vi "Puncta_fit.vi"() -> ()   [LabVIEW 2012]
uses:
  <vilib>/Utility/file.llb/Write To Spreadsheet File (DBL).vi
panel:
  in  "Batch Fit - Interate":i32=2
  in  "Reverse Order?":bool=TRUE
  in  "Single Fit":bool
  in  "Transfer to Save Buffer":bool
  out "Save Buffer":dbl[][](array[numeric])
  in  "Inverse Image?":bool=TRUE
  in  "initial parameters":dbl[](array[numeric])=[200.0, 100.0, 10.0, 10.0, 5.0, 5.0, 0.0]
  in  "Flip Width/Length?":bool=TRUE
  out "XY Fits":dbl[][](array[numeric])
  out "range fit":dbl[][](array[numeric])
  in  "Slide":cluster{i16, i16, i16}(slide)={24, 31, 24} scale=0.0..173.0
  out "Array 3":u16[][][](array[numeric])
  in  "File Path":path
  in  "Data in IFD\n(small files)":bool=TRUE
  in  "last mouse":bool
  out "Last Mouse \nPosition:":cluster{"X":i32, "Y":i32}={"X"=104, "Y"=248}
  in  "Write file":bool
  out "Bead position 3":cluster{dbl[], dbl[]}[](graph)
  out "Bead position 2":cluster{dbl[], dbl[]}[](graph)
  out "volume":dbl=1098.513843481793
  in  "Batch Fit":bool
  out "y fit position":dbl=246.994904536459
  out "x fit position":dbl=104.21273484039956
  out "residue":dbl=77.56065334791303
  in  "Wait Time":u32=50
  out "XY Graph 3":cluster{dbl[], dbl[]}(graph)={[104.5005475079822, 104.5005475079822], [248.54823101222757, 248.54823101222757]}
  out "Bead position":cluster{dbl[], dbl[]}[](graph)
  in  "Load Image":bool
  out "Fit":dbl[][](graph)
  out "best fit parameters":dbl[](array[numeric])
  out "number of \nfunction calls":i32=210
  out "Data":u16[][](graph)
  out "Extracted Image":T1(plugin-control)
  in  "buffer":i16=7
  out "Image":T1(plugin-control)
  in  "Image Type":T2=7 items=["Grayscale (U8)", "Grayscale (I16)", "Grayscale (SGL)", "Complex (CSG)", "RGB (U32)", "HSL (U32)", "RGB (U64)", "Grayscale (U16)"]
  in  "stop":bool
  out "Image Pixels (U16)":u16[][](graph)
  # "Background"
  # "Amp"
  # "x"
  # "y"
  # "x s.d."
  # "y s.d."
  # "angle"
  # "y fit"
  # "x fit"
  # "Volume"
  # "x S.D."
  # "Amp"
  # "Frame"
  # "sub x"
  # "sub y"
  # "Amp"
  # "x sub fit"
  # "y sub fit"
  # "y S.D."
  # "angle"
  # "Background"
  # "This program loads a .tiff stack and then a 2D Gaussian is fit to individual puncta over multiple frames.  Previous (or future) frame is used for initial fit condition of current frame."
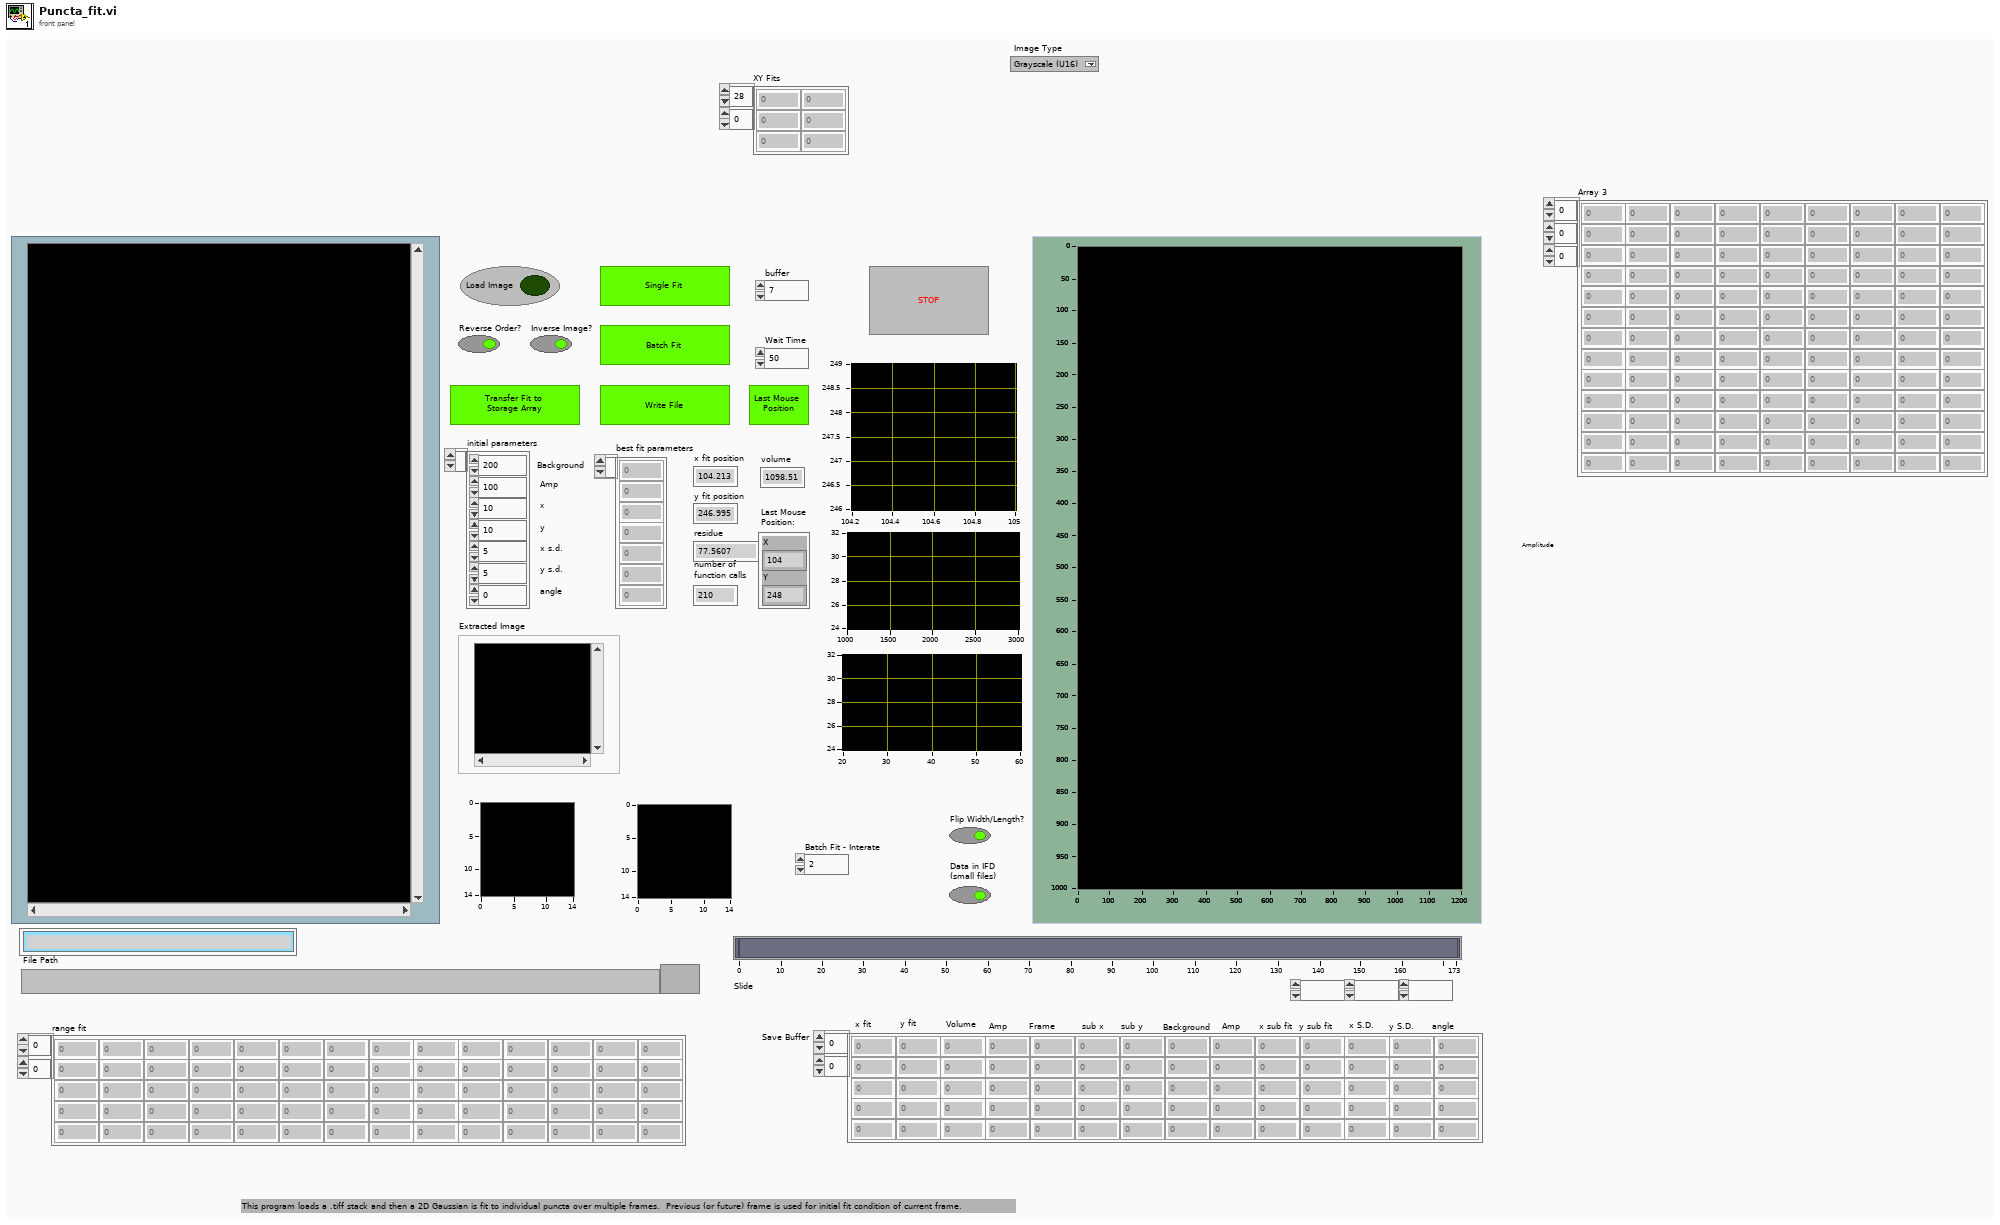
[diagram p1: front panel]
types:
  T1 = typedef "IMAQ Image.ctl" = refnum<image>
  T2 = typedef "Image Type" = u32
  T3 = cluster{"XScale.Maximum":dbl, "YScale.Maximum":dbl}
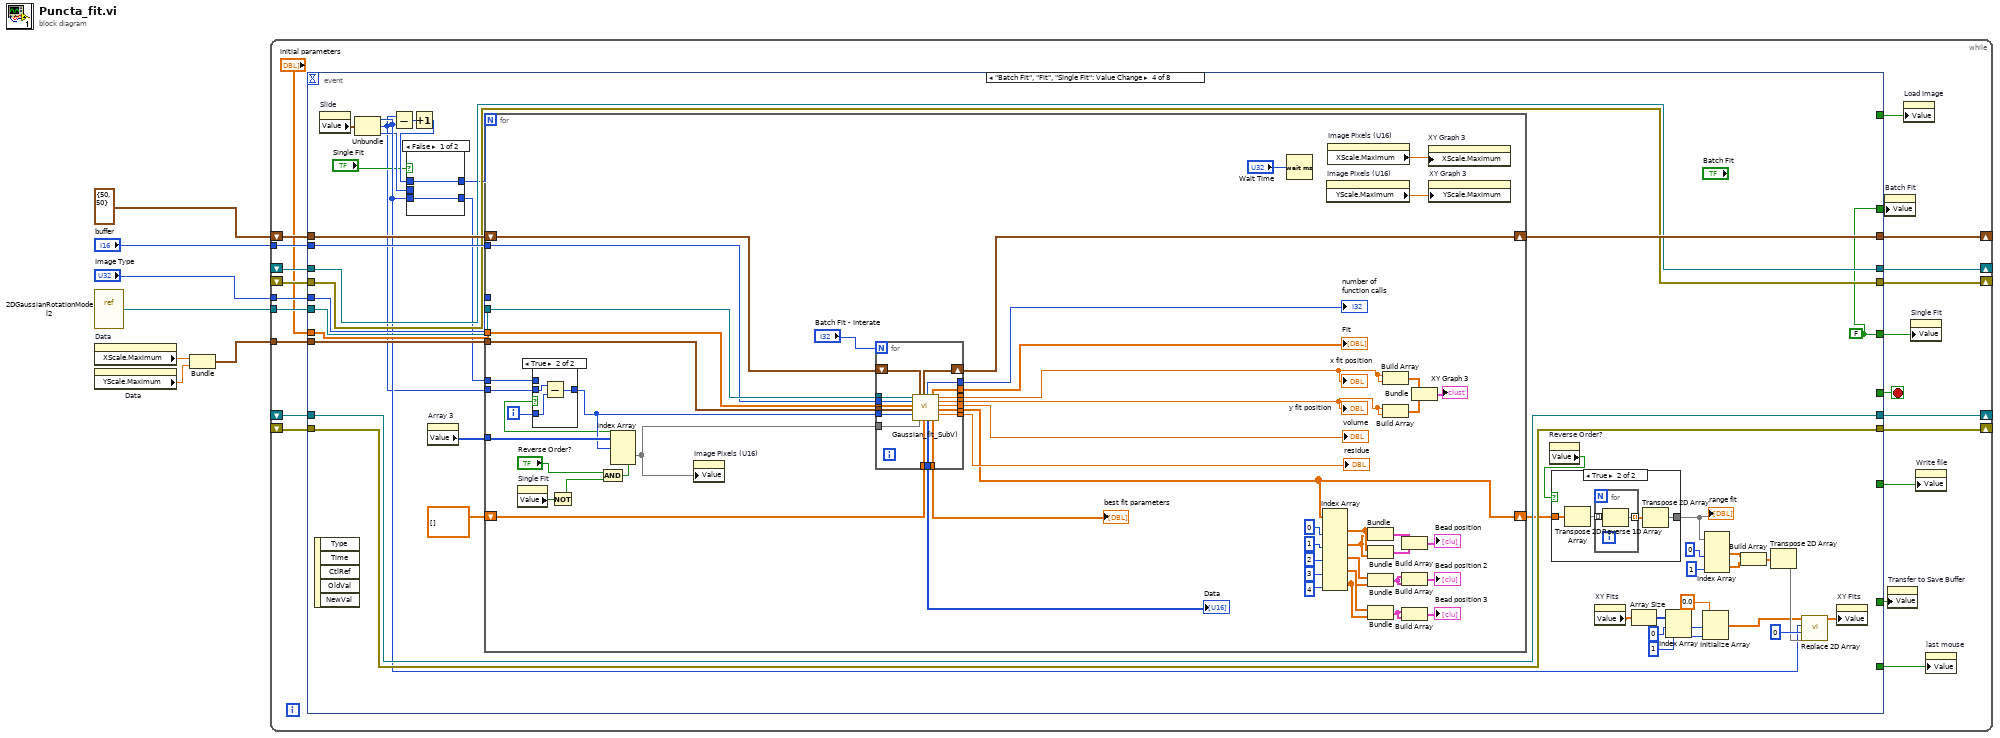
[diagram p0: block diagram]
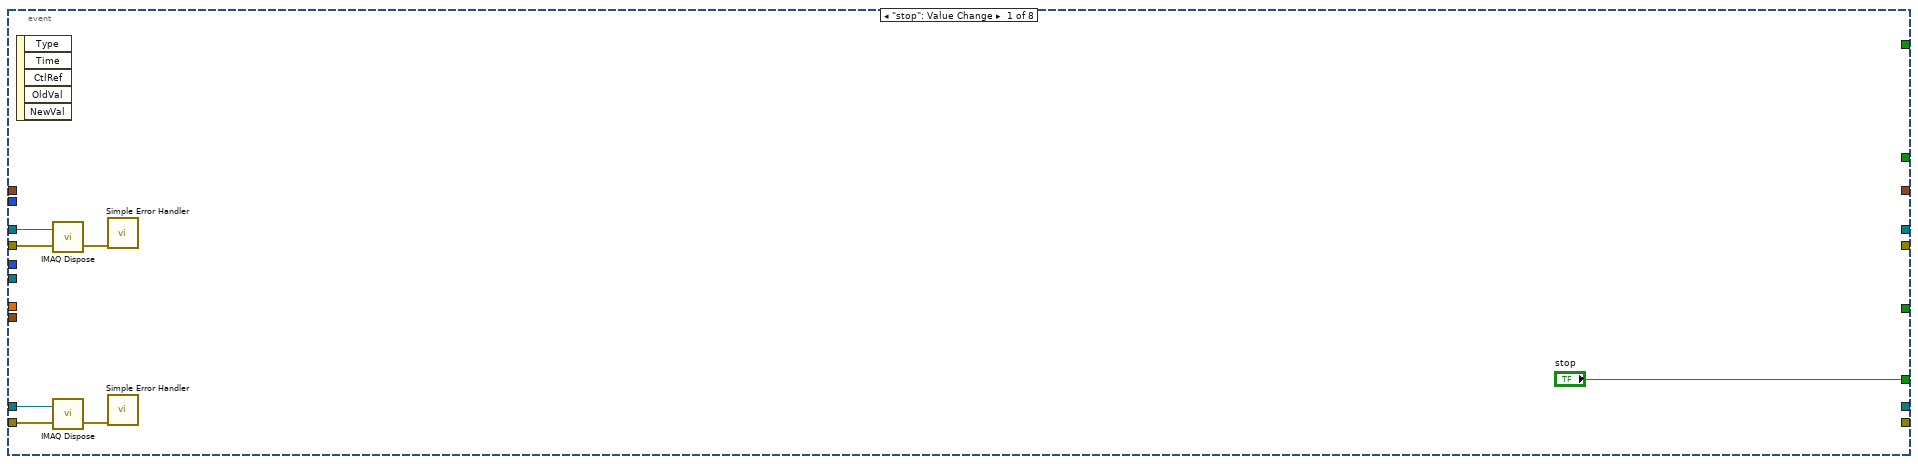
[diagram p2: hidden frame]
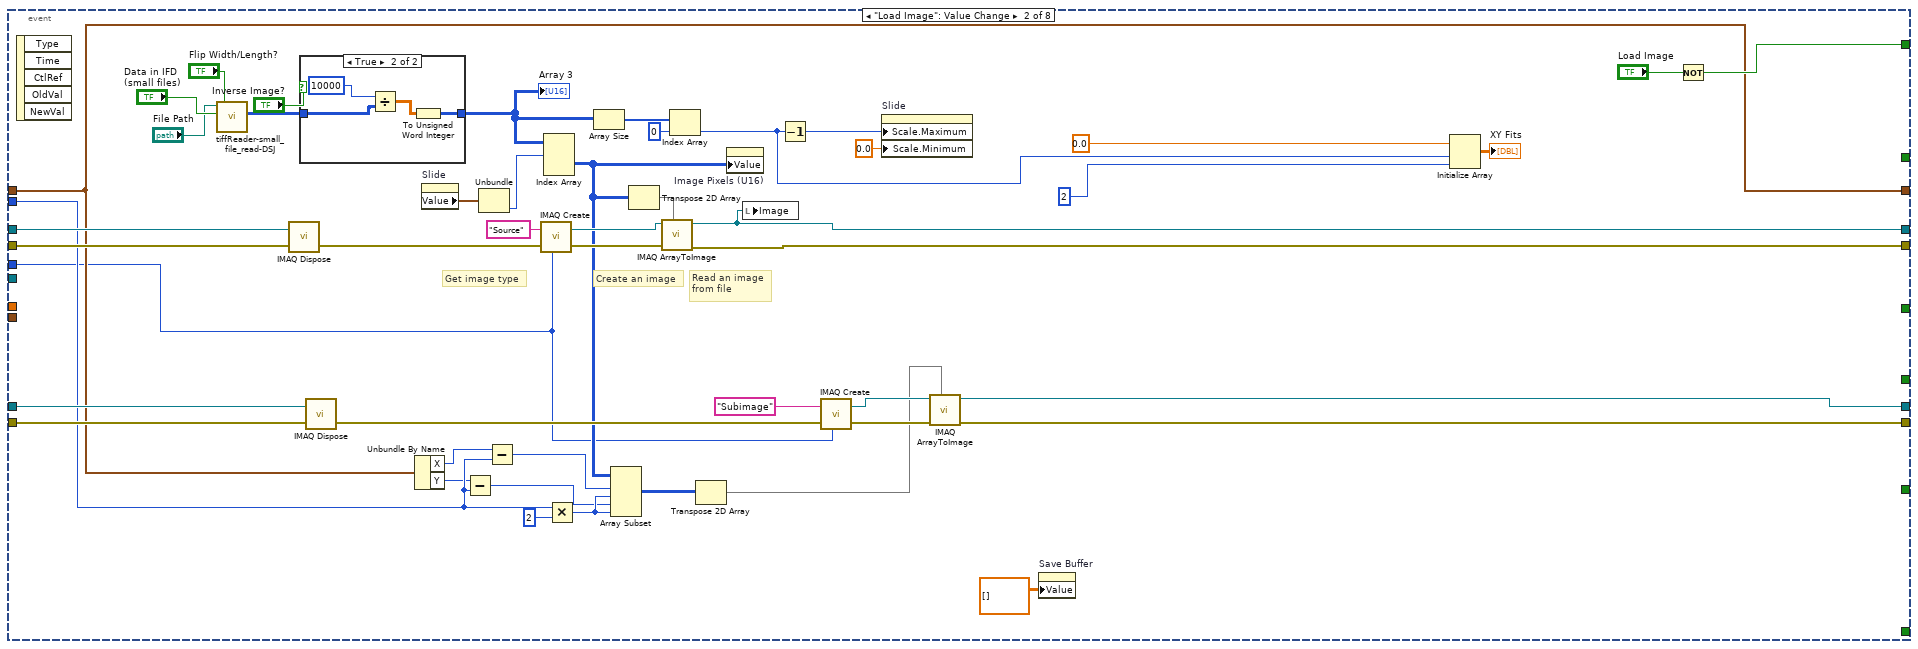
[diagram p3: hidden frame]
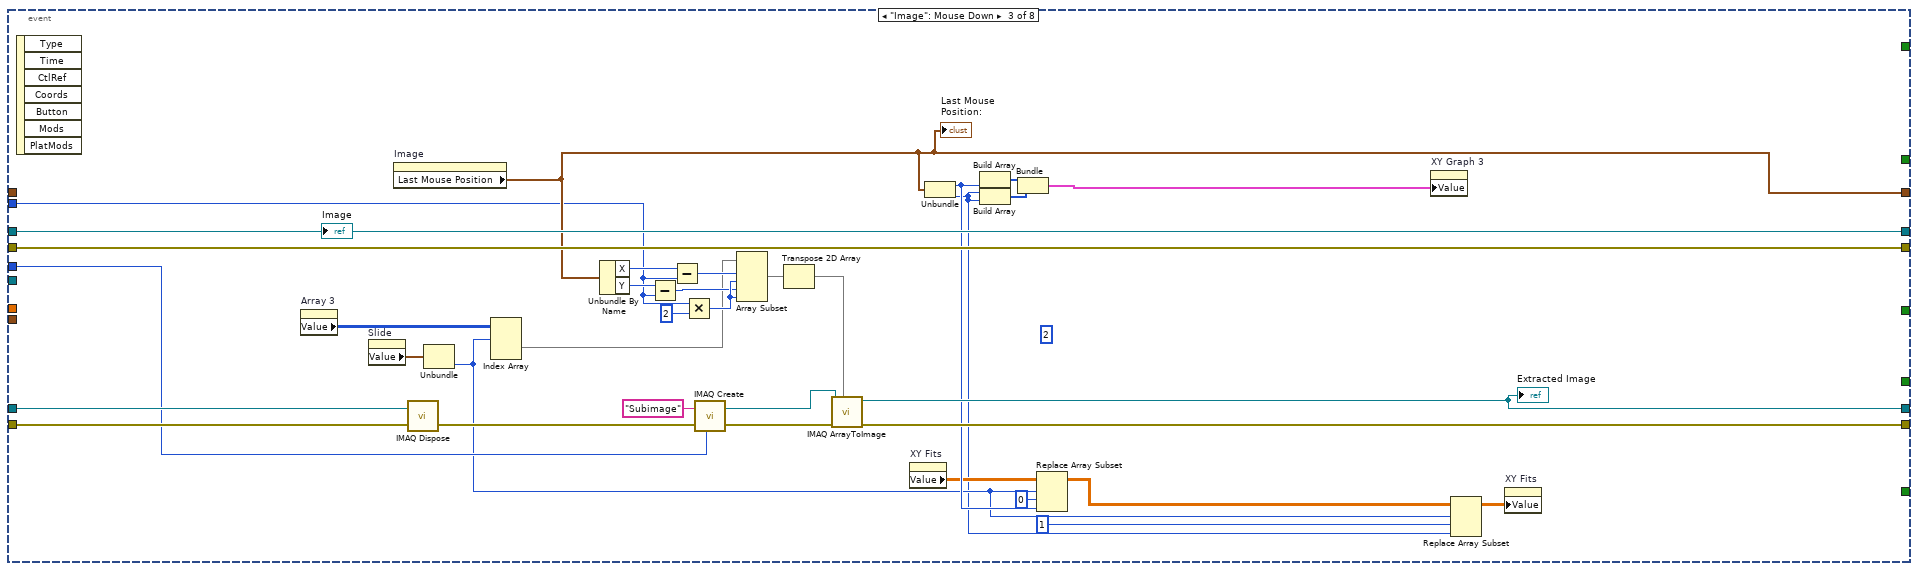
[diagram p5: hidden frame]
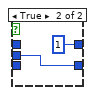
[diagram p7: hidden frame]
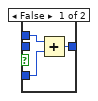
[diagram p8: hidden frame]
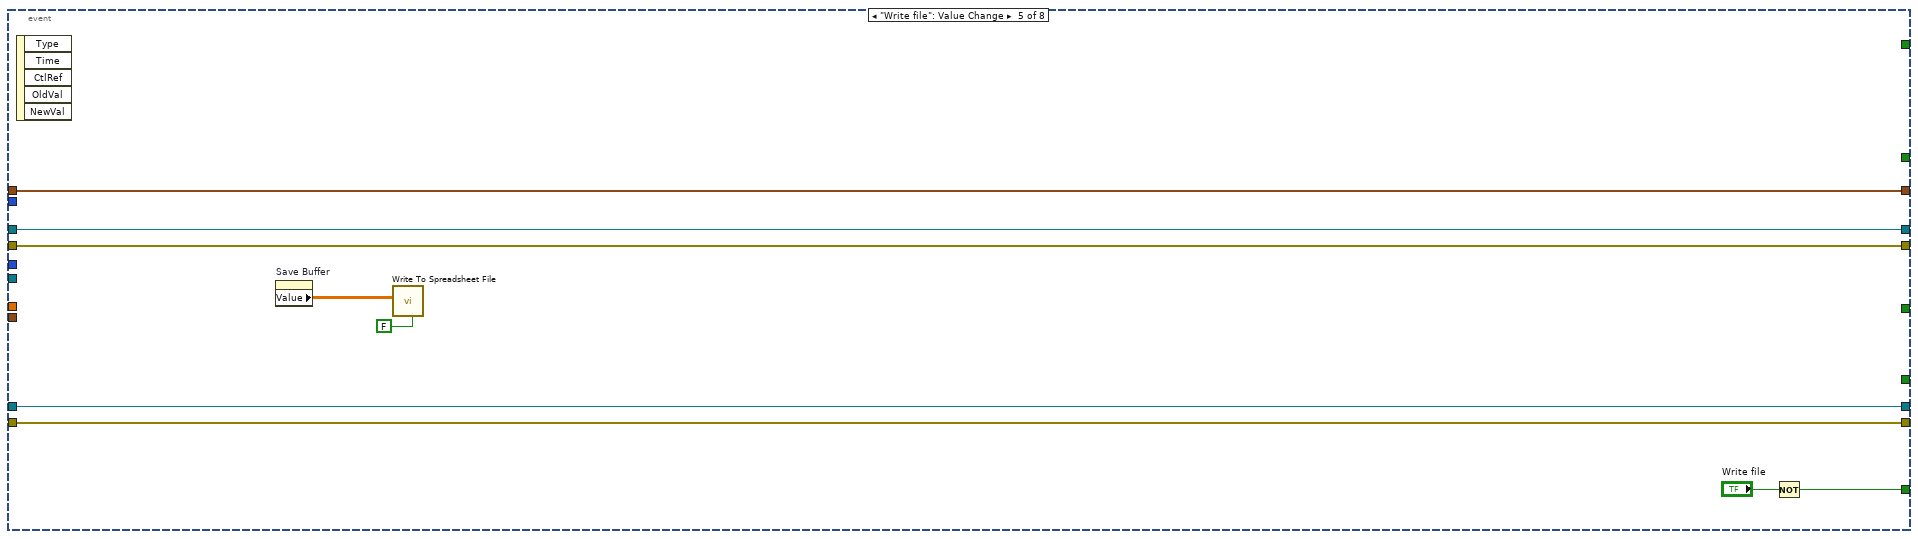
[diagram p9: hidden frame]
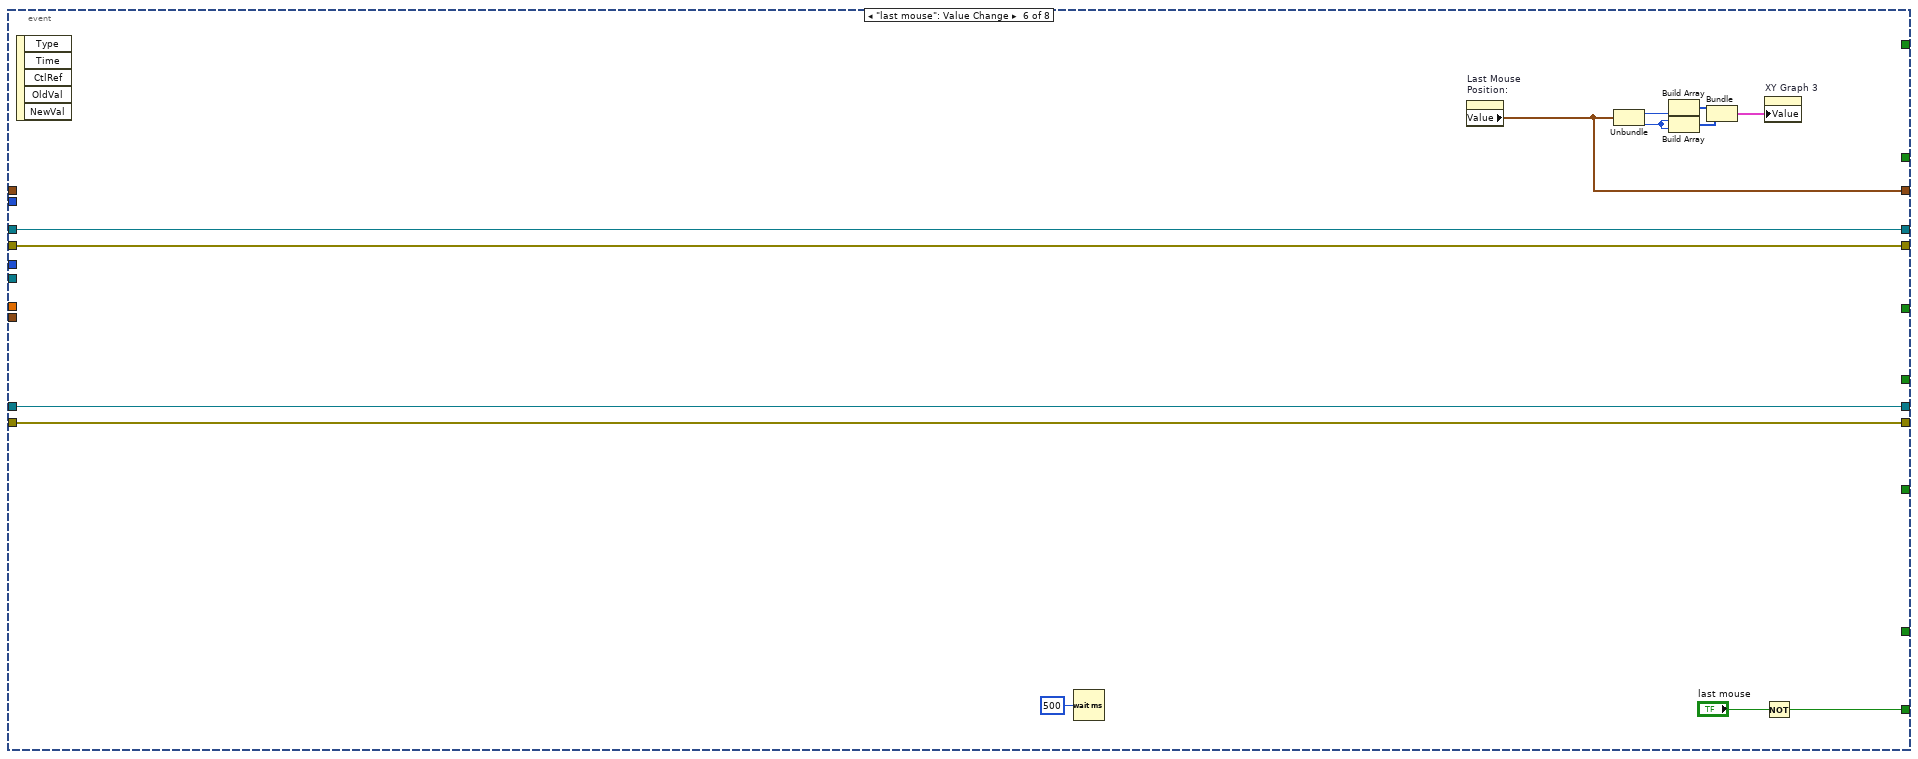
[diagram p10: hidden frame]
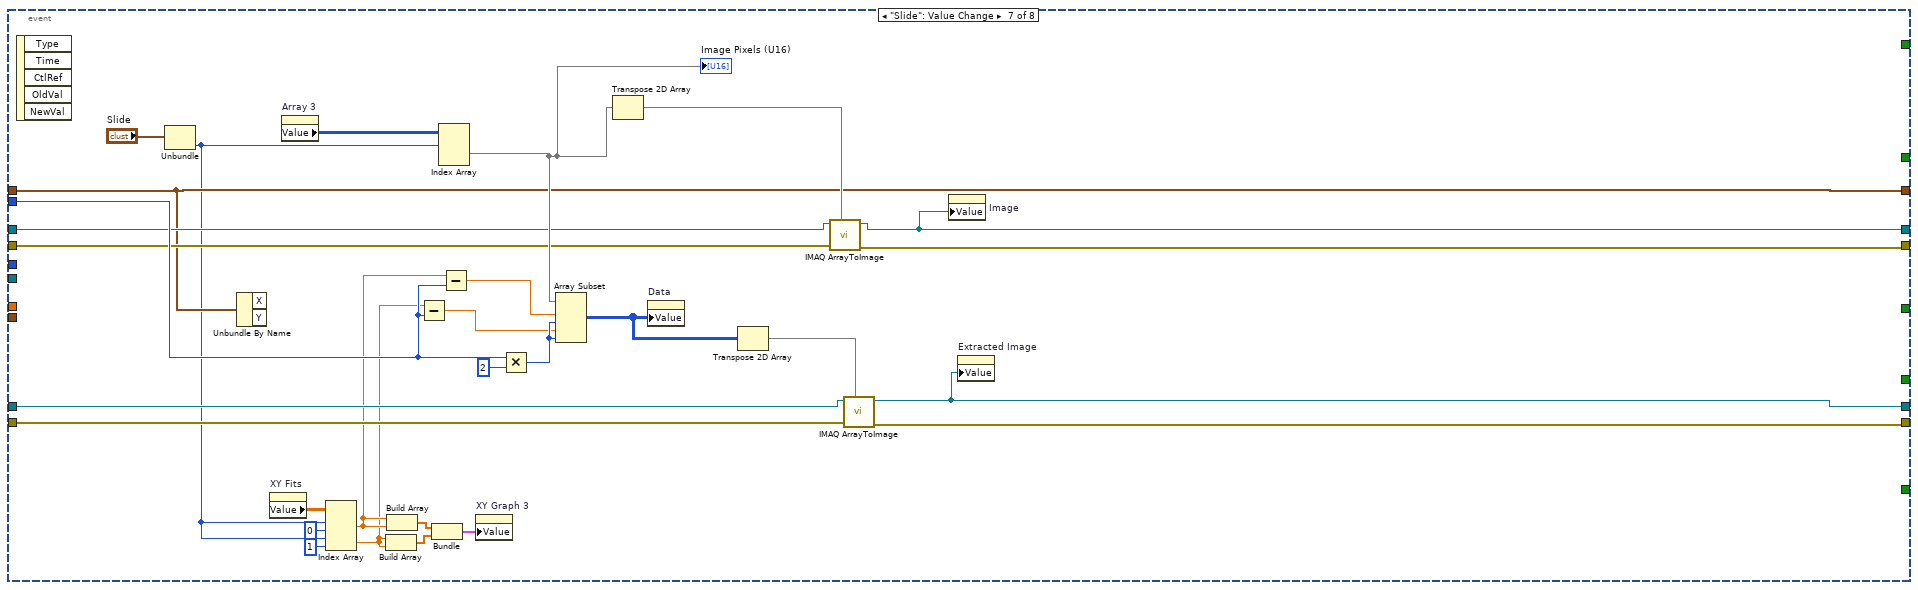
[diagram p11: hidden frame]
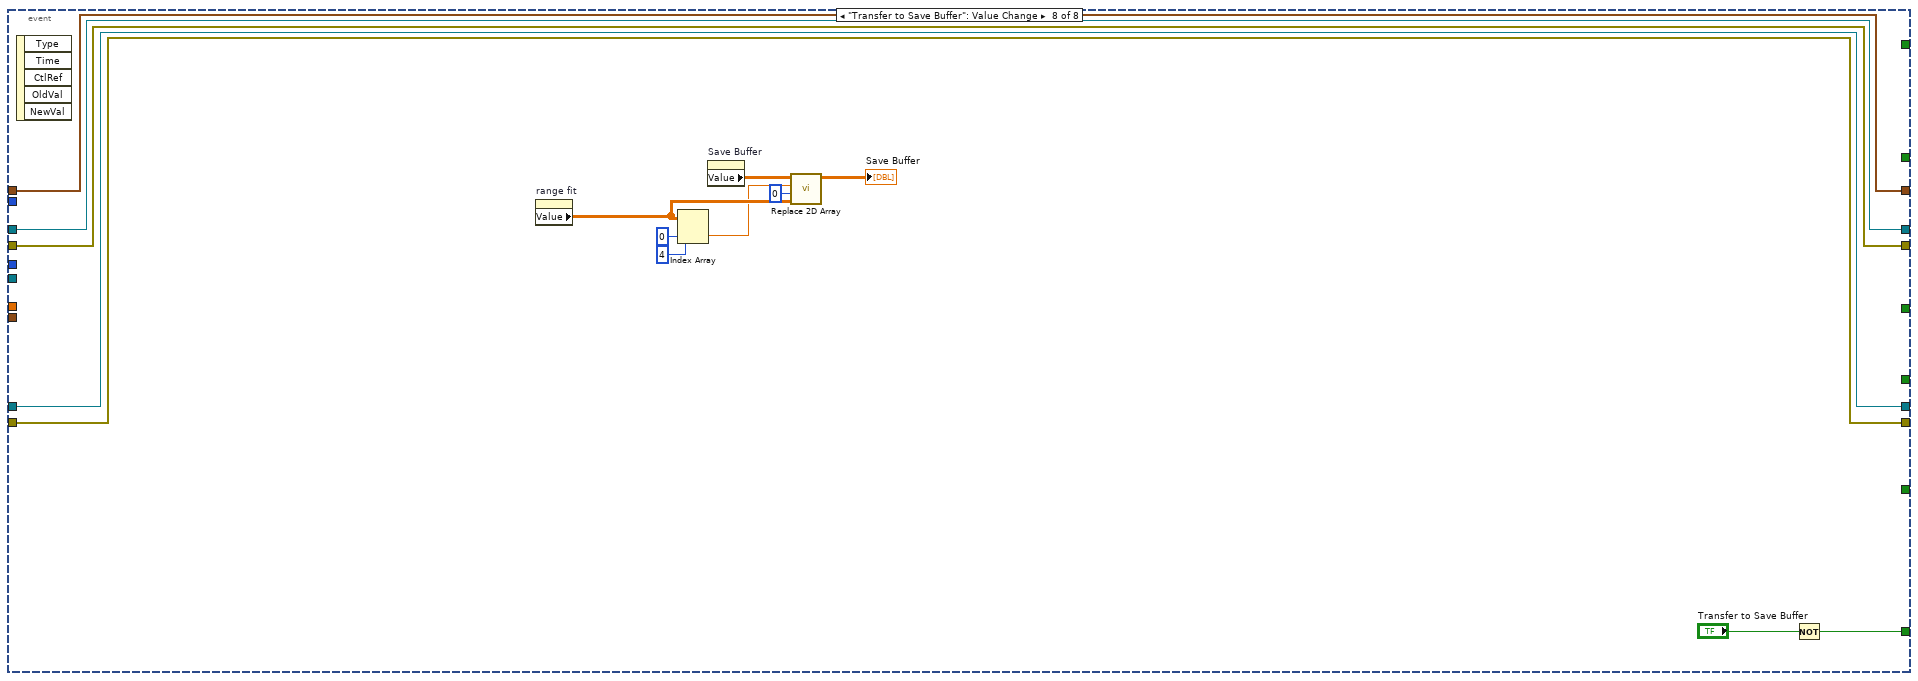
[diagram p12: hidden frame]
diagram:
  n1 = vi-ref "2DGaussianRotationModel2.vi"() -> (w7:refnum<vi>)
  n2 = property on="Data" class="IntGraph (strict)"() -> ("XScale.Maximum"=w5:dbl)  [unwired: 2 in, 2 out]
  n3 = property on="Data" class="IntGraph (strict)"() -> ("YScale.Maximum"=w4:dbl)  [unwired: 2 in, 2 out]
  n4 = Bundle("XScale.Maximum"=w5, "YScale.Maximum"=w4) -> (w6:T3)  [unwired: 1 in]
  n5 = while {
    shift-right: [w28] -> _
    shift-left: _ -> [w27]
    shift-right: [w26] -> _
    shift-left: _ -> [w25]
    shift-right: [w23] -> _
    shift-left: _ -> [w21]
    shift-right: [w24] -> _
    shift-left: _ -> [w22]
    tunnel: w7 -> [w20]
    tunnel: w6 -> [w19]
    tunnel: "buffer" -> [w17]
    shift-right: [w16] -> _
    shift-left: cluster{"X":i32, "Y":i32} {"X"=50, "Y"=50} ("Value") -> [w15]
    tunnel: "Image Type" -> [w14]
    stop <- w29 stop-if-true
    n6 = event shown="[3] \"Batch Fit\", \"Fit\", \"Single Fit\": Value Change" {
      selector: _ -> [_ _ _ _ _ _ _ _]
      dyn-events: _ -> [_ _ _ _ _ _ _ _]
      timeout: _ -> [_ _ _ _ _ _ _ _]
      tunnel: ["stop" _ _ _ _ _ _ _] -> w29
      tunnel: w27 -> [w35 w82 w123 w159 w259 w273 w288 w315]
      tunnel: [_ w76 w123 w159 w259 w273 w300 w315] -> w28
      tunnel: [_ w73 w124 w158 w258 w270 w302 w314] -> w26
      tunnel: w25 -> [w34 w83 w124 w158 w258 w270 w289 w314]
      tunnel: [_ w48 w102 w155 w257 w272 w299 w313] -> w24
      tunnel: [_ w49 w103 w157 w256 w271 w301 w312] -> w23
      tunnel: w22 -> [w32 w67 w122 w155 w257 w272 w287 w313]
      tunnel: w21 -> [w31 w66 w121 w157 w256 w271 w286 w312]
      tunnel: w20 -> [_ _ _ w163 _ _ _ _]
      tunnel: w19 -> [_ _ _ w165 _ _ _ _]
      tunnel: [_ w80 _ _ _ _ _ _] -> w18
      tunnel: w17 -> [_ w56 w107 w160 _ _ w292 _]
      tunnel: [_ w57 w108 w166 w260 w263 w283 w316] -> w16
      tunnel: w15 -> [_ w57 _ w161 w260 _ w283 w316]
      tunnel: "initial parameters" -> [_ _ _ w164 _ _ _ _]
      tunnel: [_ _ _ w130 _ _ _ _] -> w13
      tunnel: w14 -> [_ w53 w118 w162 _ _ _ _]
      tunnel: [_ _ _ _ w254 _ _ _] -> w12
      tunnel: [_ _ _ _ _ w268 _ _] -> w11
      tunnel: [_ _ _ _ _ _ _ w304] -> w9
      tunnel: [_ _ _ w130 _ _ _ _] -> w8
      event "stop": Value Change {
        n7 = event-data() -> ()  [unwired: 1 in, 5 out]
        n8 = call "IMAQ Dispose"("Image"=w35, "error in (no error)"=w34) -> ("error out"=w33:errorcluster)  [unwired: 1 in, 3 out]
        n9 = call "IMAQ Dispose"("Image"=w32, "error in (no error)"=w31) -> ("error out"=w30:errorcluster)  [unwired: 1 in, 3 out]
        n10 = call <vilib>:"Simple Error Handler.vi"("error in (no error)"=w33) -> ()  [unwired: 1 in, 8 out]
        n11 = call <vilib>:"Simple Error Handler.vi"("error in (no error)"=w30) -> ()  [unwired: 1 in, 8 out]
      }
      event "Load Image": Value Change {
        # "Get image type"
        # "Read an image\nfrom file"
        # "Create an image"
        n12 = event-data() -> ()  [unwired: 1 in, 5 out]
        n13 = call "tiffReader-small_file_read-DSJ.vi"("Flip Width/Length?"="Flip Width/Length?", "Data in IFD\n(small files)"="Data in IFD\n(small files)", "File Path"="File Path") -> ("Array 3"=w40:u16[][][])  [unwired: 1 in, 3 out]
        n14 = call "IMAQ Dispose"("Image"=w82, "error in (no error)"=w83) -> ("error out"=w79:errorcluster)  [unwired: 1 in, 3 out]
        n15 = case shown="True" "Inverse Image?" {
          tunnel: w40 -> [w85 w89]
          tunnel: [w85 w86] -> w39
          frame False {
          }
          frame True {
            n16 = Divide(x=10000 ("dimension size"), y=w89) -> (x/y=w87:dbl[][][])
            n17 = To Unsigned Word Integer(number=w87) -> (unsigned 16bit integer=w86:u16[][][])
          }
        }
        "Array 3" <- w39
        n18 = call "IMAQ Dispose"("Image"=w67, "error in (no error)"=w66) -> ("error out"=w59:errorcluster)  [unwired: 1 in, 3 out]
        n19 = Unbundle By Name(w57) -> ("X"=w45:i32, "Y"=w44:i32)
        n20 = property on="Slide" class="Slide (strict)"() -> ("Value"=w65:cluster{i16, i16, i16})  [unwired: 2 in, 2 out]
        n21 = Subtract(x=w44, y=w56) -> (x-y=w61:i32)
        n22 = Unbundle(w65) -> (w64:i16)  [unwired: 2 out]
        n23 = Subtract(x=w45, y=w56) -> (x-y=w60:i32)
        n24 = call "IMAQ Create"("Image Name"="Source", "Image Type"=w53, "error in (no error)"=w79) -> ("New Image"=w75:T1, "error out"=w74:errorcluster)  [unwired: 1 in, 1 out]
        n25 = Index Array(array=w39, index (dim 0)=w64) -> (element=w58:u16[][])  [unwired: 2 in]
        n26 = Multiply(x=w56, y=i16 2) -> (x*y=w62:i16)
        n27 = Array Size(array=w39) -> (size(s)=w71:i32[])
        n28 = Array Subset(array=w58, index (row)=w60, length (row)=w62, index (col)=w61, length (col)=w62) -> (w55:u16[][])
        n29 = Transpose 2D Array(2D array=w58) -> (transposed array=w72:u16[][])
        n30 = call "IMAQ ArrayToImage"("Image Pixels (U16)"=w72, "error in (no error)"=w74, "Image"=w75) -> ("error out"=w73:errorcluster, "Image Out"=w76:T1)  [unwired: 7 in]
        n31 = Index Array(array=w71, index=0) -> (element=w43:i32)
        n32 = Transpose 2D Array(2D array=w55) -> (transposed array=w50:u16[][])
        n33 = property on="Image Pixels (U16)" class="IntGraph (strict)"("Value"=w58) -> ()  [unwired: 2 in, 2 out]
        n34 = local write "Image"(w76) -> ()
        n35 = Decrement(x=w43) -> (x-1=w68:i32)
        n36 = call "IMAQ Create"("Image Name"="Subimage", "Image Type"=w53, "error in (no error)"=w59) -> ("New Image"=w52:T1, "error out"=w51:errorcluster)  [unwired: 1 in, 1 out]
        n37 = property on="Slide" class="Slide (strict)"("Scale.Maximum"=w68, "Scale.Minimum"=0.0 ("Scale.Range:Minimum")) -> ()  [unwired: 2 in, 2 out]
        n38 = call "IMAQ ArrayToImage"("Image Pixels (U16)"=w50, "error in (no error)"=w51, "Image"=w52) -> ("error out"=w49:errorcluster, "Image Out"=w48:T1)  [unwired: 7 in]
        n39 = property on="Save Buffer" class="Arr (strict)"("Value"=dbl[][] [] ("Save Buffer")) -> ()  [unwired: 2 in, 2 out]
        n40 = Initialize Array(0.0 ("element"), w43, 2 ("dimension size")) -> (→"XY Fits":dbl[][])
        n41 = Not(x="Load Image") -> (.not. x?=w80:bool)
      }
      event "Image": Mouse Down {
        (unwired) 2 ("dimension size")
        n42 = event-data() -> ()  [unwired: 1 in, 7 out]
        n43 = property on="Array 3" class="Arr (strict)"() -> ("Value"=w98:u16[][][])  [unwired: 2 in, 2 out]
        n44 = property on="Slide" class="Slide (strict)"() -> ("Value"=w106:cluster{i16, i16, i16})  [unwired: 2 in, 2 out]
        n45 = property on="Image" class="ImageControl"() -> ("Last Mouse Position"=w108:cluster{"X":i32, "Y":i32})  [unwired: 2 in, 2 out]
        "Last Mouse \nPosition:" <- w108
        n46 = call "IMAQ Dispose"("Image"=w122, "error in (no error)"=w121) -> ("error out"=w120:errorcluster)  [unwired: 1 in, 3 out]
        n47 = Unbundle(w106) -> (w94:i16)  [unwired: 2 out]
        n48 = Index Array(array=w98, index (dim 0)=w94) -> (element=w105:u16[][])  [unwired: 2 in]
        n49 = Unbundle By Name(w108) -> ("X"=w109:i32, "Y"=w110:i32)
        n50 = Subtract(x=w110, y=w107) -> (x-y=w112:i32)
        n51 = Subtract(x=w109, y=w107) -> (x-y=w111:i32)
        n52 = Multiply(x=w107, y=i16 2) -> (x*y=w113:i16)
        n53 = call "IMAQ Create"("Image Name"="Subimage", "Image Type"=w118, "error in (no error)"=w120) -> ("New Image"=w101:T1, "error out"=w104:errorcluster)  [unwired: 1 in, 1 out]
        n54 = Array Subset(array=w105, index (row)=w111, length (row)=w113, index (col)=w112, length (col)=w113) -> (w100:u16[][])
        n55 = Transpose 2D Array(2D array=w100) -> (transposed array=w99:u16[][])
        n56 = call "IMAQ ArrayToImage"("Image Pixels (U16)"=w99, "error in (no error)"=w104, "Image"=w101) -> ("error out"=w103:errorcluster, "Image Out"=w102:T1)  [unwired: 7 in]
        "Extracted Image" <- w102
        n57 = property on="XY Fits" class="Arr (strict)"() -> ("Value"=w95:dbl[][])  [unwired: 2 in, 2 out]
        n58 = Unbundle(w108) -> ("X"=w96:i32, "Y"=w92:i32)
        n59 = Build Array(w96, w96) -> (w117:i32[])
        n60 = Build Array(w92, w92) -> (w116:i32[])
        n61 = Bundle(w117, w116) -> (w115:cluster{i32[], i32[]})  [unwired: 1 in]
        n62 = Replace Array Subset(array=w95, new element=w96, index (row)=w94, index (col)=0 ("disabled index (col)")) -> (w91:dbl[][])
        n63 = property on="XY Graph 3" class="XYGraph (strict)"("Value"=w115) -> ()  [unwired: 2 in, 2 out]
        n64 = Replace Array Subset(array=w91, new element=w92, index (row)=w94, index (col)=1 ("disabled index (col)")) -> (w90:dbl[][])
        n65 = property on="XY Fits" class="Arr (strict)"("Value"=w90) -> ()  [unwired: 2 in, 2 out]
        "Image" <- w123
      }
      event "Batch Fit", "Fit", "Single Fit": Value Change {
        w130 = FALSE ("Fit!")
        n66 = event-data() -> ()  [unwired: 1 in, 5 out]
        n67 = property on="Slide" class="Slide (strict)"() -> ("Value"=w154:cluster{i16, i16, i16})  [unwired: 2 in, 2 out]
        n68 = Unbundle(w154) -> (w134:i16, w129:i16, w132:i16)
        n69 = Subtract(x=w129, y=w134) -> (x-y=w153:i16)
        n70 = Increment(x=w153) -> (x+1=w135:i16)
        n71 = case shown="False" "Single Fit" {
          tunnel: [w175 i16 1 ("y")] -> w136
          tunnel: w135 -> [w175 _]
          tunnel: w134 -> [w174 _]
          tunnel: [w174 w176] -> w133
          tunnel: w132 -> [_ w176]
          frame False {
          }
          frame True {
          }
        }
        n72 = property on="Array 3" class="Arr (strict)"() -> ("Value"=w156:u16[][][])  [unwired: 2 in, 2 out]
        n73 = for {
          N: w136 -> [_]
          shift-right: [w225] -> w166
          shift-left: w161 -> [w224]
          tunnel: w160 -> [w208]
          tunnel: w163 -> [w227]
          tunnel: w164 -> [w226]
          tunnel: w165 -> [w223]
          tunnel: w162 -> [_]
          tunnel: w156 -> [w207]
          tunnel: w133 -> [w205]
          shift-right: [w199] -> w127
          shift-left: dbl[][] [] -> [w200]
          tunnel: w129 -> [w183]
          i -> [w204]
          n74 = property on="Single Fit" class="Bool (strict)"() -> ("Value"=w182:bool)  [unwired: 2 in, 2 out]
          n75 = Not(x=w182) -> (.not. x?=w181:bool)
          n76 = And(x="Reverse Order?", y=w181) -> (x .and. y?=w179:bool)
          n77 = case shown="True" w179 {
            tunnel: w205 -> [w248 _]
            tunnel: w204 -> [w247 w251]
            tunnel: [w246 w249] -> w201
            tunnel: w183 -> [_ w250]
            frame False {
              n78 = Add(x=w248, y=w247) -> (x+y=w246:i32)
            }
            frame True {
              n79 = Subtract(x=w250, y=w251) -> (x-y=w249:i32)
            }
          }
          n80 = Index Array(array=w207, index (dim 0)=w201) -> (element=w206:u16[][])  [unwired: 2 in]
          n81 = property on="Image Pixels (U16)" class="IntGraph (strict)"("Value"=w206) -> ()  [unwired: 2 in, 2 out]
          n82 = for {
            N: "Batch Fit - Interate" -> [_]
            tunnel: w227 -> [w245]
            tunnel: w226 -> [w244]
            tunnel: w223 -> [w241]
            tunnel: [w240] -> w216
            tunnel: w208 -> [w239]
            tunnel: w206 -> [w238]
            tunnel: [w237] -> w203
            tunnel: [w236] -> w202
            tunnel: w201 -> [w235]
            tunnel: w200 -> [w234]
            tunnel: [w233] -> w199
            tunnel: [w232] -> w188
            tunnel: [w231] -> w187
            tunnel: [w230] -> w186
            tunnel: [w229] -> w185
            tunnel: [w228] -> w184
            shift-right: [w243] -> w225
            shift-left: w224 -> [w242]
            n83 = call "Gaussian_fit_SubV).vi"("Fit model"=w245, "sub array buffer"=w239, "initial parameters"=w244, "Cluster"=w241, "Image Index"=w235, "Fit position"=w242, "Image Array"=w238, "Array 3"=w234) -> ("Value 3"=w243:cluster{"X":i32, "Y":i32}, "number of function calls"=w232:i32, "Array"=w228:u16[][], "best nonlinear fit"=w231:dbl[][], "best fit parameters"=w229:dbl[], "Numeric 4"=w237:dbl, "Numeric 3"=w236:dbl, "Numeric out"=w230:dbl, "Array 2"=w233:dbl[][], "residue"=w240:dbl)  [unwired: 2 in]
          }
          "residue" <- w216
          "x fit position" <- w203
          "y fit position" <- w202
          "number of \nfunction calls" <- w188
          "Fit" <- w187
          "volume" <- w186
          "best fit parameters" <- w185
          "Data" <- w184
          n84 = Wait (ms)(milliseconds to wait="Wait Time") -> ()  [unwired: 1 out]
          n85 = Index Array(array=w199, index (col) #1=0 ("index (row)"), index (col) #2=1 ("index (row)"), index (col) #3=2 ("index (row)"), index (col) #4=3 ("index (row)"), index (col) #5=4 ("index (row)")) -> (element #1=w198:dbl[], element #2=w197:dbl[], element #3=w196:dbl[], element #4=w195:dbl[], element #5=w194:dbl[])  [unwired: 5 in]
          n86 = property on="Image Pixels (U16)" class="IntGraph (strict)"() -> ("YScale.Maximum"=w219:dbl)  [unwired: 2 in, 2 out]
          n87 = property on="Image Pixels (U16)" class="IntGraph (strict)"() -> ("XScale.Maximum"=w218:dbl)  [unwired: 2 in, 2 out]
          n88 = Bundle("Array 2"=w198, "Array 2"=w197) -> (w214:cluster{"Array 2":dbl[], "Array 2":dbl[]})  [unwired: 1 in]
          n89 = Bundle("Array 2"=w198, "Array 2"=w197) -> (w215:cluster{"Array 2":dbl[], "Array 2":dbl[]})  [unwired: 1 in]
          n90 = Bundle("Array 2"=w196, "Array 2"=w194) -> (w212:cluster{"Array 2":dbl[], "Array 2":dbl[]})  [unwired: 1 in]
          n91 = Bundle("Array 2"=w195, "Array 2"=w194) -> (w210:cluster{"Array 2":dbl[], "Array 2":dbl[]})  [unwired: 1 in]
          n92 = Build Array(w203, w203) -> (w222:dbl[])
          n93 = Build Array(w202, w202) -> (w221:dbl[])
          n94 = Build Array(w214, w215) -> (→"Bead position":cluster{"Array 2":dbl[], "Array 2":dbl[]}[])
          n95 = Build Array(w212, w212) -> (→"Bead position 2":cluster{"Array 2":dbl[], "Array 2":dbl[]}[])
          n96 = Build Array(w210, w210) -> (→"Bead position 3":cluster{"Array 2":dbl[], "Array 2":dbl[]}[])
          n97 = Bundle(w222, w221) -> (→"XY Graph 3":cluster{dbl[], dbl[]})  [unwired: 1 in]
          n98 = property on="XY Graph 3" class="XYGraph (strict)"("XScale.Maximum"=w218) -> ()  [unwired: 2 in, 2 out]
          n99 = property on="XY Graph 3" class="XYGraph (strict)"("YScale.Maximum"=w219) -> ()  [unwired: 2 in, 2 out]
        }
        n100 = property on="Reverse Order?" class="Bool (strict)"() -> ("Value"=w125:bool)  [unwired: 2 in, 2 out]
        n101 = case shown="True" w125 {
          tunnel: w127 -> [w167 w169]
          tunnel: [w167 w168] -> w126
          frame False {
          }
          frame True {
            n102 = Transpose 2D Array(2D array=w169) -> (transposed array=w170:dbl[][])
            n103 = for {
              tunnel: w170 -> [w173] mode=indexing
              tunnel: [w172] -> w171 mode=indexing
              n104 = Reverse 1D Array(array=w173) -> (reversed array=w172:dbl[])
            }
            n105 = Transpose 2D Array(2D array=w171) -> (transposed array=w168:dbl[][])
          }
        }
        "range fit" <- w126
        n106 = property on="XY Fits" class="Arr (strict)"() -> ("Value"=w143:dbl[][])  [unwired: 2 in, 2 out]
        n107 = Array Size(array=w143) -> (size(s)=w142:i32[])
        n108 = Index Array(array=w142, index #1=0 ("index"), index #2=1 ("index")) -> (element #1=w139:i32, element #2=w138:i32)
        n109 = Initialize Array(0.0 ("element"), w139, w138) -> (w128:dbl[][])
        n110 = Index Array(array=w126, index (col) #1=0 ("disabled index (row)"), index (col) #2=1 ("index (col)")) -> (element #1=w149:dbl[], element #2=w148:dbl[])  [unwired: 2 in]
        n111 = Build Array(w149, w148) -> (w145:dbl[][])
        n112 = Transpose 2D Array(2D array=w145) -> (transposed array=w144:dbl[][])
        n113 = call "Replace 2D Array.vi"("Elements to Replace"=w144, "Replacement Column"=0 ("Replacement Row"), "Replacement Row"=w134, "Current Array"=w128) -> ("output array"=w147:dbl[][])  [unwired: 7 in]
        n114 = property on="XY Fits" class="Arr (strict)"("Value"=w147) -> ()  [unwired: 2 in, 2 out]
      }
      event "Write file": Value Change {
        n115 = event-data() -> ()  [unwired: 1 in, 5 out]
        n116 = property on="Save Buffer" class="Arr (strict)"() -> ("Value"=w252:dbl[][])  [unwired: 2 in, 2 out]
        n117 = call-poly <vilib>:"Write To Spreadsheet File.vi"("transpose? (no:F)"=FALSE, "2D data"=w252) -> ()  [unwired: 6 in, 1 out]
        n118 = Not(x="Write file") -> (.not. x?=w254:bool)
      }
      event "last mouse": Value Change {
        n119 = event-data() -> ()  [unwired: 1 in, 5 out]
        n120 = Wait (ms)(milliseconds to wait=u32 500) -> ()  [unwired: 1 out]
        n121 = property on="Last Mouse \nPosition:" class="Clust (strict)"() -> ("Value"=w263:cluster{"X":i32, "Y":i32})  [unwired: 2 in, 2 out]
        n122 = Unbundle(w263) -> ("X"=w262:i32, "Y"=w261:i32)
        n123 = Build Array(w262, w262) -> (w266:i32[])
        n124 = Build Array(w261, w261) -> (w265:i32[])
        n125 = Bundle(w266, w265) -> (w264:cluster{i32[], i32[]})  [unwired: 1 in]
        n126 = Not(x="last mouse") -> (.not. x?=w268:bool)
        n127 = property on="XY Graph 3" class="XYGraph (strict)"("Value"=w264) -> ()  [unwired: 2 in, 2 out]
      }
      event "Slide": Value Change {
        n128 = event-data() -> ()  [unwired: 1 in, 5 out]
        n129 = Unbundle("Slide") -> (w278:i16)  [unwired: 2 out]
        n130 = Unbundle By Name(w283) -> ()  [unwired: 2 out]
        n131 = property on="XY Fits" class="Arr (strict)"() -> ("Value"=w279:dbl[][])  [unwired: 2 in, 2 out]
        n132 = property on="Array 3" class="Arr (strict)"() -> ("Value"=w298:u16[][][])  [unwired: 2 in, 2 out]
        n133 = Index Array(array=w279, index (row) #1=w278, index (col) #1=0 ("disabled index (col)"), index (row) #2=w278, index (col) #2=1 ("disabled index (col)")) -> (element #1=w275:dbl, element #2=w274:dbl)
        n134 = Build Array(w274, w274) -> (w282:dbl[])
        n135 = Build Array(w275, w275) -> (w281:dbl[])
        n136 = Subtract(x=w274, y=w292) -> (x-y=w294:dbl)
        n137 = Bundle(w281, w282) -> (w280:cluster{dbl[], dbl[]})  [unwired: 1 in]
        n138 = Index Array(array=w298, index (dim 0)=w278) -> (element=w290:u16[][])  [unwired: 2 in]
        "Image Pixels (U16)" <- w290
        n139 = Subtract(x=w275, y=w292) -> (x-y=w293:dbl)
        n140 = property on="XY Graph 3" class="XYGraph (strict)"("Value"=w280) -> ()  [unwired: 2 in, 2 out]
        n141 = Multiply(x=w292, y=i16 2) -> (x*y=w295:i16)
        n142 = Array Subset(array=w290, index (row)=w293, length (row)=w295, index (col)=w294, length (col)=w295) -> (w285:u16[][])
        n143 = Transpose 2D Array(2D array=w290) -> (transposed array=w291:u16[][])
        n144 = property on="Data" class="IntGraph (strict)"("Value"=w285) -> ()  [unwired: 2 in, 2 out]
        n145 = Transpose 2D Array(2D array=w285) -> (transposed array=w284:u16[][])
        n146 = call "IMAQ ArrayToImage"("Image Pixels (U16)"=w291, "error in (no error)"=w289, "Image"=w288) -> ("error out"=w302:errorcluster, "Image Out"=w300:T1)  [unwired: 7 in]
        n147 = call "IMAQ ArrayToImage"("Image Pixels (U16)"=w284, "error in (no error)"=w286, "Image"=w287) -> ("error out"=w301:errorcluster, "Image Out"=w299:T1)  [unwired: 7 in]
        n148 = property on="Image" class="ImageControl"("Value"=w300) -> ()  [unwired: 2 in, 2 out]
        n149 = property on="Extracted Image" class="ImageControl"("Value"=w299) -> ()  [unwired: 2 in, 2 out]
      }
      event "Transfer to Save Buffer": Value Change {
        n150 = event-data() -> ()  [unwired: 1 in, 5 out]
        n151 = property on="range fit" class="Arr (strict)"() -> ("Value"=w307:dbl[][])  [unwired: 2 in, 2 out]
        n152 = Index Array(array=w307, index (row)=0, index (col)=4 ("disabled index (col)")) -> (element=w303:dbl)
        n153 = property on="Save Buffer" class="Arr (strict)"() -> ("Value"=w309:dbl[][])  [unwired: 2 in, 2 out]
        n154 = call "Replace 2D Array.vi"("Elements to Replace"=w307, "Replacement Column"=0, "Replacement Row"=w303, "Current Array"=w309) -> ("output array"=→"Save Buffer":dbl[][])  [unwired: 7 in]
        n155 = Not(x="Transfer to Save Buffer") -> (.not. x?=w304:bool)
      }
    }
    n156 = property on="Batch Fit" class="Bool (strict)"("Value"=w13) -> ()  [unwired: 2 in, 2 out]
    n157 = property on="Transfer to Save Buffer" class="Bool (strict)"("Value"=w9) -> ()  [unwired: 2 in, 2 out]
    n158 = property on="Load Image" class="Bool (strict)"("Value"=w18) -> ()  [unwired: 2 in, 2 out]
    n159 = property on="Single Fit" class="Bool (strict)"("Value"=w8) -> ()  [unwired: 2 in, 2 out]
    n160 = property on="Write file" class="Bool (strict)"("Value"=w12) -> ()  [unwired: 2 in, 2 out]
    n161 = property on="last mouse" class="Bool (strict)"("Value"=w11) -> ()  [unwired: 2 in, 2 out]
  }
